vi "CC.vi"(10 "AD":T2={"电压最大值"=10013, " 电压最小值"=10013, " 采样率"=10013, "每通道采样率"=10013, "采样模式"=10123, "接线方式"=10106, "source"="OnboardClock", "选择通道AD "="USB_6211_2/ai1"} {"采样模式" items=["有限采样"=10178, "连续采样"=10123, "硬件定时单点"=12522]; "接线方式" items=["默认"=-1, "RSE"=10083, "NRSE"=10078, "差分"=10106, "伪差分"=12529]}, 11 "DA":T1={"电压最大值"=0.0, " 电压最小值"=0.0, "选择通道DA "="USB_6211_2/ao1"}) -> (0 "error out":errorcluster caption="错误输出", 3 "prodatascan":T3)   [LabVIEW 2018]
uses:
  Setting/AD.ctl
  Setting/DA.ctl
  ProData/prodatascan.ctl
  <vilib>/DAQmx/read.llb/DAQmx Read (Analog 1D DBL 1Chan NSamp).vi
  <vilib>/DAQmx/write.llb/DAQmx Write (Analog DBL 1Chan 1Samp).vi
  <vilib>/DAQmx/create/channels.llb/DAQmx Create Channel (AI-Voltage-Basic).vi
  <vilib>/DAQmx/configure/timing.llb/DAQmx Timing (Sample Clock).vi
  <vilib>/DAQmx/create/channels.llb/DAQmx Create Channel (AO-Voltage-Basic).vi
  <vilib>/DAQmx/miscellaneous.llb/DAQmx Fill In Error Info.vi
panel:
  out "AD6211":tag
  out "nVpai":dbl
  out "minindex":i32
  out "maxindex":i32
  out "min":dbl
  out "max":dbl
  out "ScanOut":dbl(graph)
  out "while get stop":bool
  in  "freeCounter":i32=3
  out "free":dbl(graph)
  in  "扫描步进值":dbl=0.005
  out "扫描数据量":dbl
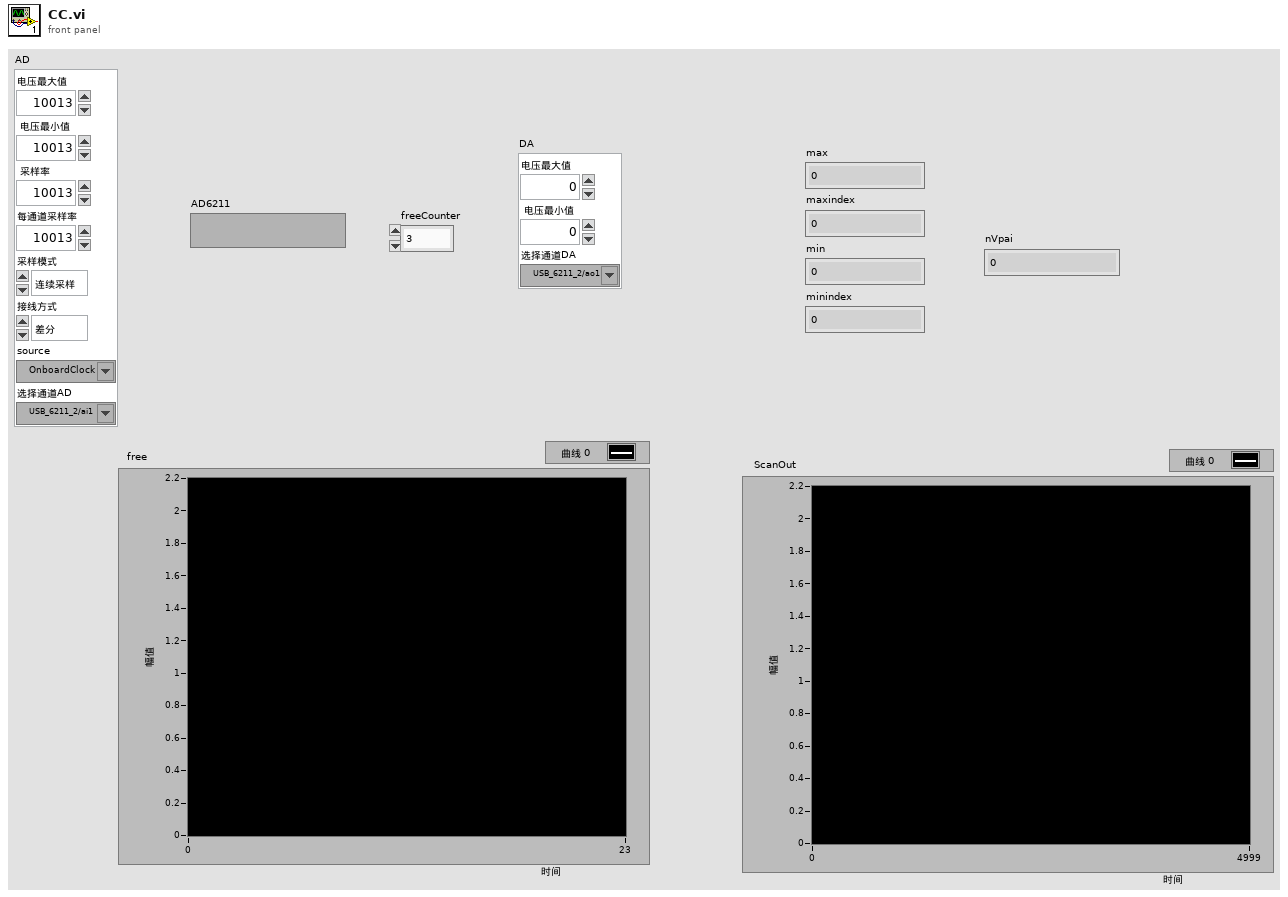
[diagram p1: front panel]
types:
  T1 = typedef "DA.ctl" = cluster{"电压最大值":dbl, " 电压最小值":dbl, "选择通道DA ":tag}
  T2 = typedef "AD.ctl" = cluster{"电压最大值":u16, " 电压最小值":i16, " 采样率":u16, "每通道采样率":u16, "采样模式":i32, "接线方式":i32, "source":tag, "选择通道AD ":tag}
  T3 = cluster{"max":dbl, "min":dbl, " nvpai":dbl, "初始化数组":dbl[]}
  T4 = typedef "prodatascan.ctl" = cluster{"max":dbl, "min":dbl, " nvpai":dbl, "初始化数组":dbl[]}
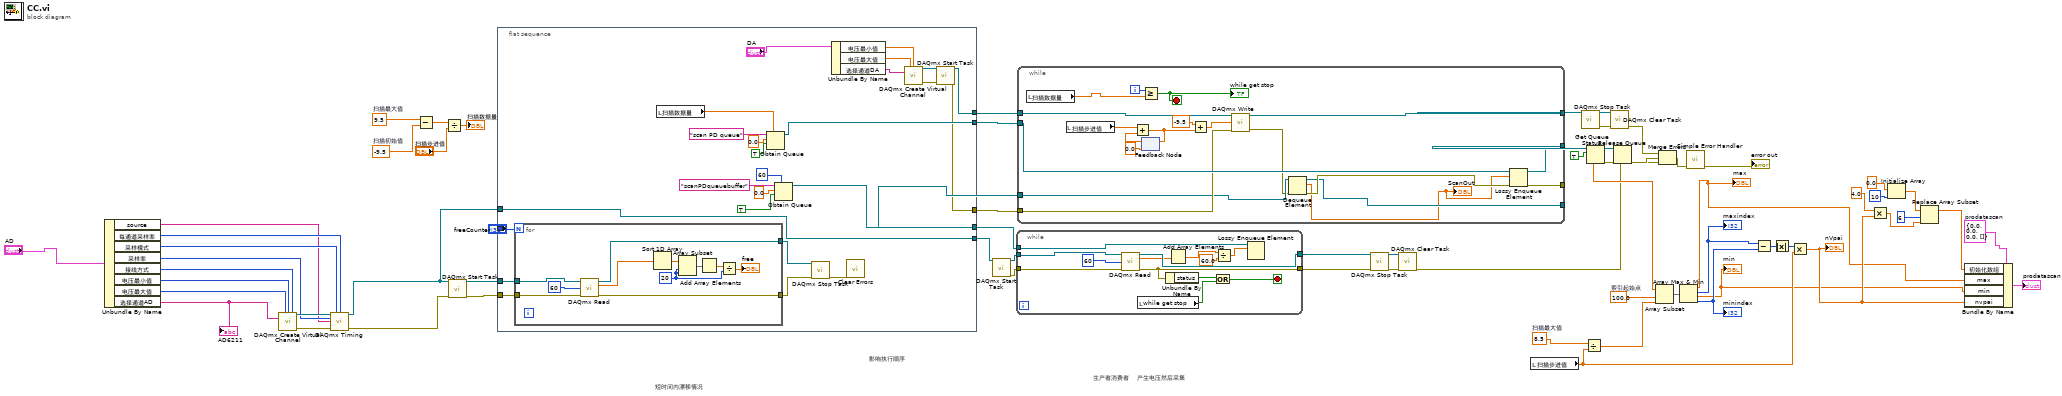
[diagram p0: block diagram]
diagram:
  w7 = T4 {"max"=0.0, "min"=0.0, " nvpai"=0.0, "初始化数组"=[]}  # prodatascan
  w38 = 100.0  # 索引起始点
  w37 = 8.5  # 扫描最大值
  w64 = 9.5  # 扫描最大值
  w65 = -9.5  # 扫描初始值
  # "生产者消费者    产生电压然后采集"
  # "影响执行顺序"
  # "短时间内漂移情况"
  n1 = Unbundle By Name("AD") -> ("source"=w21:tag, "每通道采样率"=w22:u16, "采样模式"=w23:i32, "采样率"=w24:u16, "接线方式"=w30:i32, "电压最小值"=w25:i16, "电压最大值"=w26:u16, "选择通道AD"=w27:tag)
  "AD6211" <- w27
  n2 = call-poly <vilib>:"DAQmx Create Virtual Channel.vi"("maximum value"=w26, "minimum value"=w25, "input terminal configuration"=w30, "physical channels"=w27) -> ("task out"=w29:refnum<k21>, "error out"=w28:errorcluster)  [unwired: 10 in]
  n3 = call-poly <vilib>:"DAQmx Timing.vi"("task/channels in"=w29, "sample mode"=w23, "samples per channel"=w22, "rate"=w24, "source"=w21, "error in"=w28) -> ("task out"=w2:refnum<k21>, "error out"=w20:errorcluster)  [unwired: 8 in]
  n4 = Subtract(x=w64, y=w65) -> (x-y=w66:dbl)
  n5 = Divide(x=w66, y="扫描步进值") -> (x/y=→"扫描数据量":dbl)
  n6 = call <vilib>:"DAQmx Start Task.vi"("task/channels in"=w2, "error in"=w20) -> ("task out"=w59:refnum<k21>, "error out"=w60:errorcluster)  [unwired: 12 in]
  n7 = flat-sequence {
    tunnel: "freeCounter" -> [w91]
    tunnel: w60 -> [w90]
    tunnel: w59 -> [w89]
    tunnel: [w78] -> w54
    tunnel: [w77] -> w53
    tunnel: [w76] -> w52
    tunnel: [w69] -> w5
    tunnel: w2 -> [w67]
    tunnel: [w67] -> w1
    frame #0 {
      n8 = for {
        N: w91 -> [_]
        tunnel: w89 -> [w96]
        tunnel: w90 -> [w95]
        tunnel: [w94] -> w70
        tunnel: [w93] -> w71
        w101 = 20 ("索引")
        n9 = call-poly <vilib>:"DAQmx Read.vi"("task/channels in"=w96, "number of samples per channel"=60, "error in"=w95) -> ("task out"=w94:refnum<k21>, "data"=w97:dbl[], "error out"=w93:errorcluster)  [unwired: 10 in]
        n10 = Sort 1D Array(array=w97) -> (sorted array=w102:dbl[])
        n11 = Array Subset(array=w102, index=w101, length=w101) -> (w100:dbl[])
        n12 = Add Array Elements(numeric array=w100) -> (sum=w99:dbl)
        n13 = Divide(x=w99, y=w101) -> (x/y=→"free":dbl)
      }
      n14 = local read "扫描数据量"() -> (w79:dbl)
      n15 = Obtain Queue(max queue size (-1, unlimited)=w79, name (unnamed)="scan PD queue" ("名称（未命名）"), element data type=0.0, create if not found? (T)=TRUE ("如未找到则创建？(T)")) -> (queue out=w76:refnum<queue>)  [unwired: 1 in, 2 out]
      n16 = Obtain Queue(max queue size (-1, unlimited)=60 ("队列最大值（-1，无限）"), name (unnamed)="scanPDqueuebuffer" ("名称（未命名）"), element data type=0.0, create if not found? (T)=TRUE ("如未找到则创建？(T)")) -> (queue out=w78:refnum<queue>)  [unwired: 1 in, 2 out]
      n17 = call <vilib>:"DAQmx Stop Task.vi"("task/channels in"=w70, "error in"=w71) -> ("error out"=w68:errorcluster)  [unwired: 12 in, 1 out]
      n18 = Unbundle By Name("DA") -> ("电压最小值"=w73:dbl, "电压最大值"=w74:dbl, "选择通道DA"=w75:tag)
      n19 = call <vilib>:"Clear Errors.vi"("error in (no error)"=w68) -> ()  [unwired: 5 in, 2 out]
      n20 = call-poly <vilib>:"DAQmx Create Virtual Channel.vi"("maximum value"=w74, "minimum value"=w73, "physical channels"=w75) -> ("task out"=w85:refnum<k21>, "error out"=w84:errorcluster)  [unwired: 11 in]
      n21 = call <vilib>:"DAQmx Start Task.vi"("task/channels in"=w85, "error in"=w84) -> ("task out"=w77:refnum<k21>, "error out"=w69:errorcluster)  [unwired: 12 in]
    }
  }
  n22 = call <vilib>:"DAQmx Start Task.vi"("task/channels in"=w1) -> ("task out"=w4:refnum<k21>, "error out"=w3:errorcluster)  [unwired: 13 in]
  n23 = while {
    tunnel: w3 -> [w115]
    tunnel: [w114] -> w58
    tunnel: [w113] -> w57
    tunnel: w54 -> [w110]
    tunnel: w4 -> [w108]
    stop <- w111 stop-if-true
    n24 = call-poly <vilib>:"DAQmx Read.vi"("task/channels in"=w108, "number of samples per channel"=60, "error in"=w115) -> ("task out"=w114:refnum<k21>, "data"=w105:dbl[], "error out"=w113:errorcluster)  [unwired: 10 in]
    n25 = local read "while get stop"() -> (w107:bool)
    n26 = Unbundle By Name(w113) -> ("status"=w112:bool)
    n27 = Add Array Elements(numeric array=w105) -> (sum=w104:dbl)
    n28 = Or(x=w112, y=w107) -> (x .or. y?=w111:bool)
    n29 = Divide(x=w104, y=60.0) -> (x/y=w103:dbl)
    n30 = Lossy Enqueue Element(queue=w110, element=w103) -> ()  [unwired: 1 in, 4 out]
  }
  n31 = while {
    tunnel: w54 -> [w121]
    tunnel: w53 -> [w135]
    tunnel: w52 -> [w124]
    tunnel: w5 -> [w122]
    tunnel: [w126] -> w49
    tunnel: [w125] -> _
    tunnel: [w123] -> w35
    tunnel: [w119] -> _
    i -> [w128]
    stop <- w127 stop-if-true
    n32 = local read "扫描数据量"() -> (w116:dbl)
    n33 = local read "扫描步进值"() -> (w134:dbl)
    n34 = feedback #1(0.0) -> (w132:dbl)
    n35 = Add(x=w134, y=w132) -> (x+y=w131:dbl)
    n36 = feedback-in #1(w131) -> ()
    n37 = Greater Or Equal?(x=w128, y=w116) -> (x >= y?=w127:bool)
    "while get stop" <- w127
    n38 = Add(x=-9.5, y=w131) -> (x+y=w129:dbl)
    n39 = call-poly <vilib>:"DAQmx Write.vi"("task/channels in"=w135, "data"=w129, "error in"=w122) -> ("task out"=w126:refnum<k21>, "error out"=w117:errorcluster)  [unwired: 10 in, 1 out]
    n40 = Dequeue Element(queue=w121, error in (no error)=w117) -> (queue out=w119:refnum<queue>, element=w118:dbl, error out=w120:errorcluster)  [unwired: 1 in, 1 out]
    "ScanOut" <- w118
    n41 = Lossy Enqueue Element(queue=w124, element=w118, error in (no error)=w120) -> (queue out=w123:refnum<queue>, error out=w125:errorcluster)  [unwired: 2 out]
  }
  n42 = call <vilib>:"DAQmx Stop Task.vi"("task/channels in"=w58, "error in"=w57) -> ("task out"=w55:refnum<k21>, "error out"=w56:errorcluster)  [unwired: 12 in]
  n43 = call <vilib>:"DAQmx Clear Task.vi"("task in"=w55, "error in"=w56) -> ("error out"=w31:errorcluster)  [unwired: 13 in]
  n44 = local read "扫描步进值"() -> (w36:dbl)
  n45 = call <vilib>:"DAQmx Stop Task.vi"("task/channels in"=w49) -> ("task out"=w51:refnum<k21>, "error out"=w50:errorcluster)  [unwired: 13 in]
  n46 = Divide(x=w37, y=w36) -> (x/y=w44:dbl)
  n47 = Get Queue Status(queue=w35, return elements? (F)=TRUE ("返回元素？(F)")) -> (queue out=w32:refnum<queue>, error out=w34:errorcluster, elements=w45:dbl[])  [unwired: 1 in, 5 out]
  n48 = call <vilib>:"DAQmx Clear Task.vi"("task in"=w51, "error in"=w50) -> ("error out"=w48:errorcluster)  [unwired: 13 in]
  n49 = Release Queue(queue=w32, error in (no error)=w34) -> (error out=w33:errorcluster)  [unwired: 1 in, 2 out]
  n50 = Array Subset(array=w45, index=w38, length=w44) -> (w43:dbl[])
  n51 = Merge Errors(w48, w33, w31) -> (w47:errorcluster)
  n52 = Array Max & Min(array=w43) -> (max value=w11:dbl, max index (indices)=w39:i32, min value=w10:dbl, min index (indices)=w42:i32)
  "max" <- w11
  "min" <- w10
  "maxindex" <- w39
  "minindex" <- w42
  n53 = call <vilib>:"Simple Error Handler.vi"("error in (no error)"=w47) -> ("error out"=→"error out":errorcluster)  [unwired: 4 in, 4 out]
  n54 = Subtract(x=w39, y=w42) -> (x-y=w41:i32)
  n55 = Absolute Value(x=w41) -> (abs(x)=w40:i32)
  n56 = Multiply(x=w40, y=w36) -> (x*y=w12:dbl)
  "nVpai" <- w12
  n57 = Multiply(x=4.0, y=w12) -> (x*y=w15:dbl)
  n58 = Initialize Array(0.0 ("元素"), 10 ("维数大小")) -> (w17:dbl[])
  n59 = Replace Array Subset(array=w17, new element=w15, index=6 ("索引")) -> (w14:dbl[])
  n60 = Bundle By Name(cluster=w7, "初始化数组"=w14, "max"=w11, "min"=w10, "nvpai"=w12) -> (→"prodatascan":T4)
